vi "Read_Current_values_with_slots_select.vi"(6 "error in":errorcluster, 7 "Board_index":i32[](array[numeric])=[0, 1, 2, 3], 8 "handle":i32) -> (0 "error out":errorcluster, 1 "V0Set--I0Set":T1=[[0.0, 1.0, 0.0, 1.0, 0.0, 1.0, 0.0, 1.0], [0.0, 1.0, 0.0, 1.0, 0.0, 1.0, 0.0, 1.0], [0.0, 1.0, 0.0, 1.0, 0.0, 1.0, 0.0, 1.0], [0.0, 1.0, 0.0, 1.0, 0.0, 1.0, 0.0, 1.0], [0.0, 1.0, 0.0, 1.0, 0.0, 1.0, 0.0, 1.0], [0.0, 1.0, 0.0, 1.0, 0.0, 1.0, 0.0, 1.0], [0.0, 1.0, 0.0, 1.0, 0.0, 1.0, 0.0, 1.0], [0.0, 1.0, 0.0, 1.0, 0.0, 1.0, 0.0, 1.0], [0.0, 1.0, 0.0, 1.0, 0.0, 1.0, 0.0, 1.0], [0.0, 1.0, 0.0, 1.0, 0.0, 1.0, 0.0, 1.0], [0.0, 1.0, 0.0, 1.0, 0.0, 1.0, 0.0, 1.0], [0.0, 1.0, 0.0, 1.0, 0.0, 1.0, 0.0, 1.0]], 2 "RUp--RDWn--SVMax--Trip":T1, 3 "Status":bool[][](array[boolean]), 4 "IMon--VMon":T1, 5 "Pw":bool[][](array[boolean]))   [LabVIEW 2018]
uses:
  <vilib>/Analysis/Matrix/Datatypes/RealMatrix.ctl
  <instrlib>/CAENHVWrapper/CAENHVWrapper.lvlib
  <vilib>/Analysis/Matrix/NI_Matrix.lvlib
panel:
  # "Slot 0"
  # "Slot 1"
  # "Slot 2"
  # "Slot 3"
  # "Slot 0"
  # "Slot 1"
  # "Slot 2"
  # "Slot 3"
  # "IMon"
  # "VMon"
  # "IMon"
  # "VMon"
  # "IMon"
  # "VMon"
  # "IMon"
  # "VMon"
  # "V0Set"
  # "I0Set"
  # "V0Set"
  # "I0Set"
  # "V0Set"
  # "I0Set"
  # "V0Set"
  # "I0Set"
  # "Ch 0"
  # "Slot 0"
  # "Slot 1"
  # "Slot 2"
  # "Slot 3"
  # "Slot 0"
  # "Slot 1"
  # "Slot 2"
  # "Slot 3"
  # "Ch 0"
  # "Ch 0"
  # "Ch 1"
  # "Ch 1"
  # "Ch 1"
  # "Ch 2"
  # "Ch 2"
  # "Ch 2"
  # "Ch 3"
  # "Ch 3"
  # "Ch 3"
  # "Ch 4"
  # "Ch 4"
  # "Ch 4"
  # "Ch 5"
  # "Ch 5"
  # "Ch 5"
  # "Ch 6"
  # "Ch 6"
  # "Ch 6"
  # "Ch 7"
  # "Ch 7"
  # "Ch 7"
  # "Ch 8"
  # "Ch 8"
  # "Ch 8"
  # "Ch 9"
  # "Ch 9"
  # "Ch 9"
  # "Ch 10"
  # "Ch 10"
  # "Ch 10"
  # "Ch 11"
  # "Ch 11"
  # "Ch 11"
  # "Slot 0"
  # "Slot 1"
  # "Slot 2"
  # "Slot 3"
  # "RUp"
  # "RDWn"
  # "SVMax"
  # "Trip"
  # "RUp"
  # "RDWn"
  # "SVMax"
  # "Trip"
  # "RUp"
  # "RDWn"
  # "SVMax"
  # "Trip"
  # "RUp"
  # "RDWn"
  # "SVMax"
  # "Trip"
  # "Ch 0"
  # "Ch 1"
  # "Ch 2"
  # "Ch 3"
  # "Ch 4"
  # "Ch 5"
  # "Ch 6"
  # "Ch 7"
  # "Ch 8"
  # "Ch 9"
  # "Ch 10"
  # "Ch 11"
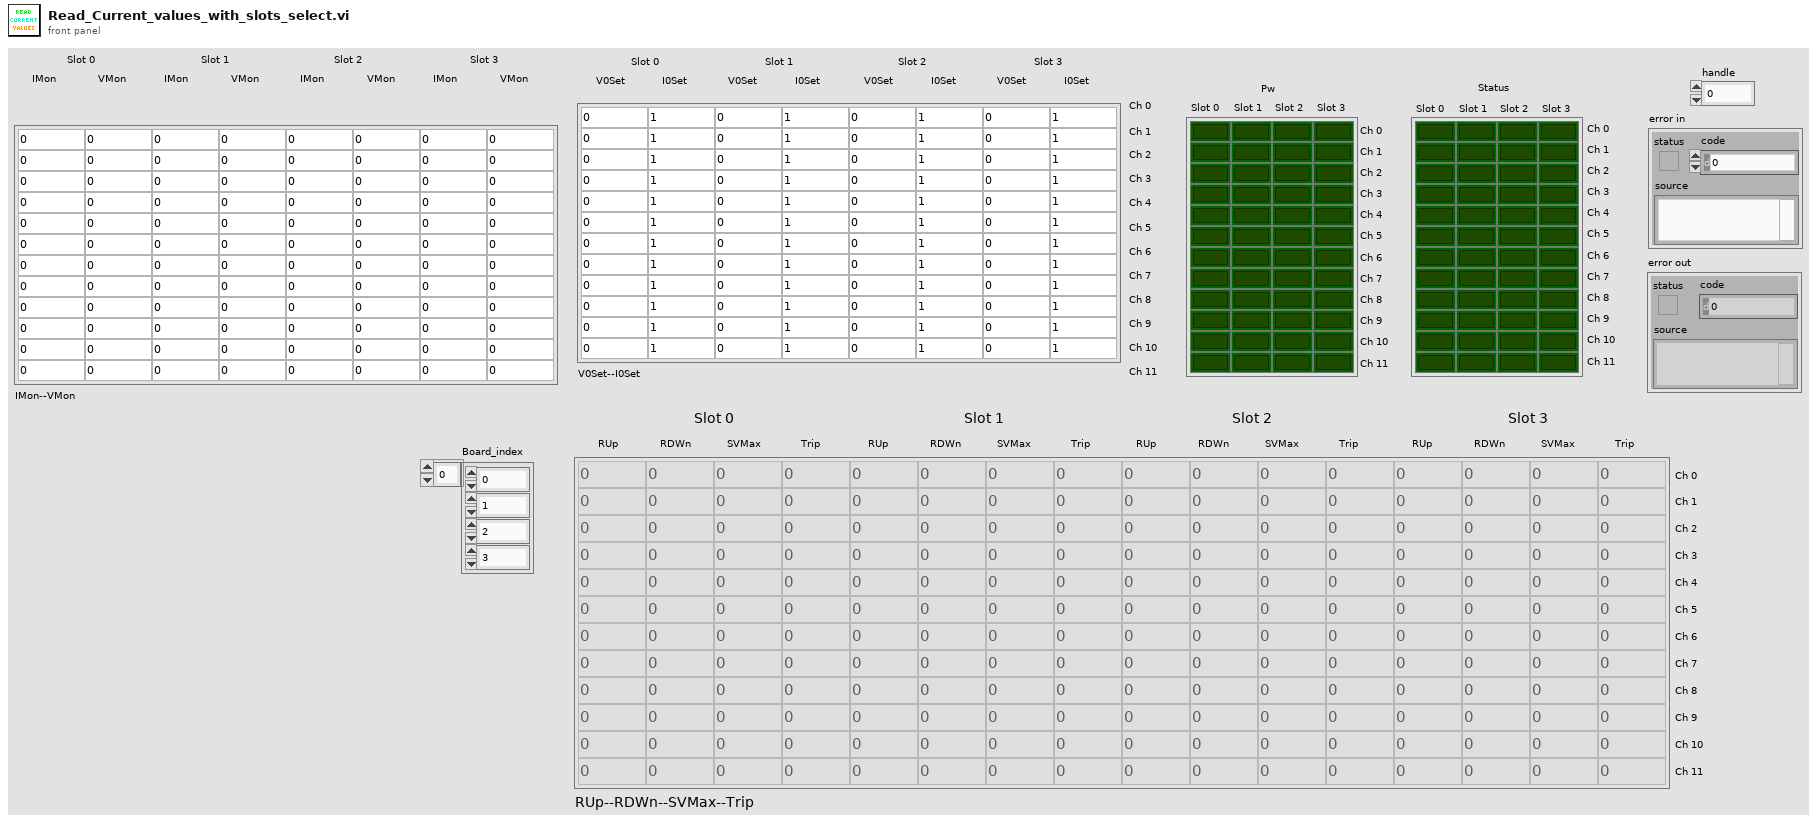
[diagram p1: front panel]
types:
  T1 = typedef "NI_Matrix.lvlib/RealMatrix.ctl" = dbl[][]
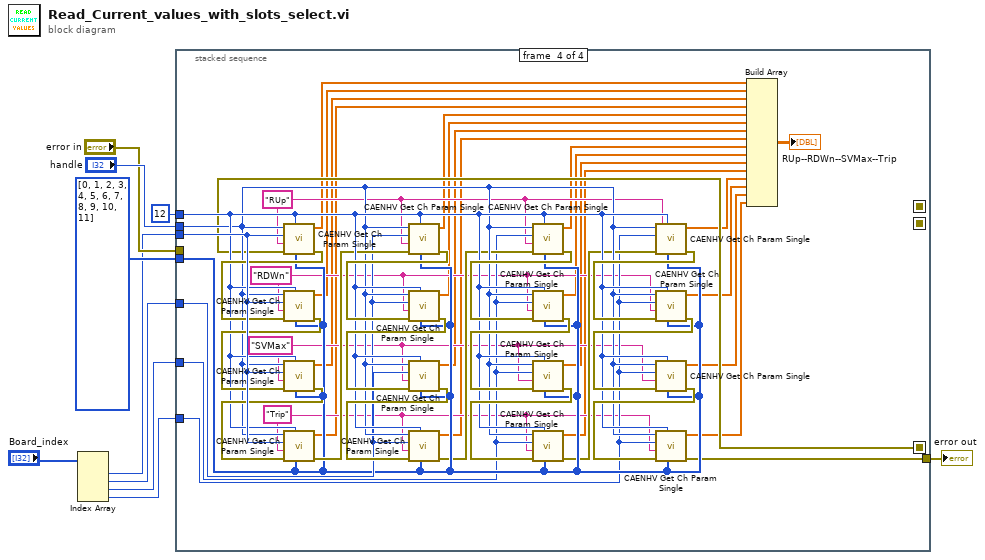
[diagram p0: block diagram]
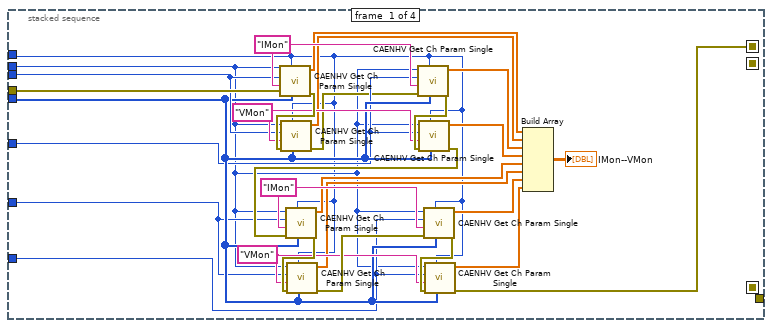
[diagram p2: hidden frame]
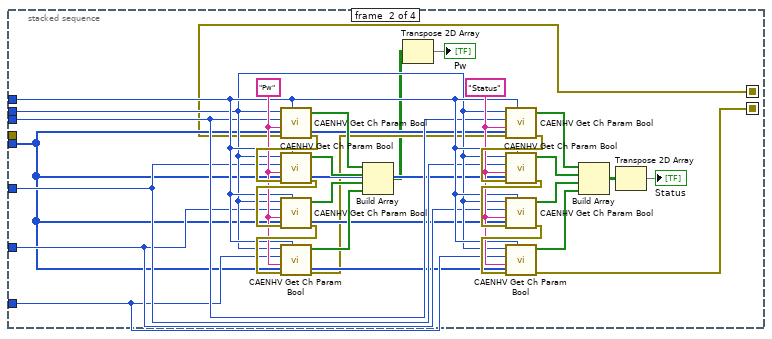
[diagram p3: hidden frame]
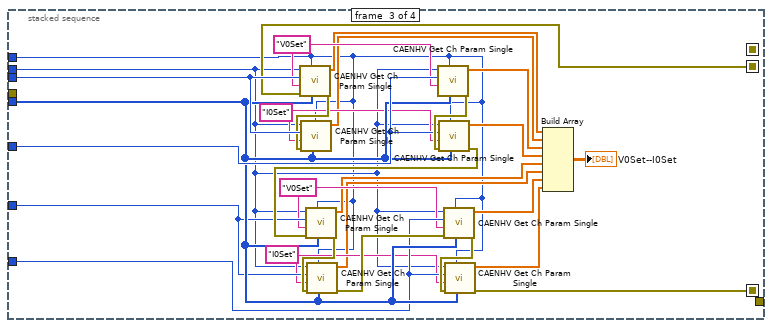
[diagram p4: hidden frame]
diagram:
  n1 = Index Array(array="Board_index") -> (element #1=w4:i32, element #2=w3:i32, element #3=w2:i32, element #4=w1:i32)  [unwired: 4 in]
  n2 = stacked-sequence {
    seq-local: [_ w45 _ _] -> [_ _ w95 _]
    seq-local: [_ _ w87 _] -> [_ _ _ w120]
    seq-local: [w14 _ _ _] -> [_ w40 _ _]
    tunnel: u16[] [0, 1, 2, 3, 4, 5, 6, 7, 8, 9, 10, 11] ("ChList") -> [w18 w47 w89 w125]
    tunnel: u16 12 ("ChNum (1)") -> [w11 w53 w70 w129]
    tunnel: "handle" -> [w12 w52 w71 w127]
    tunnel: w4 -> [w19 w51 w97 w142]
    tunnel: w3 -> [w17 w50 w93 w126]
    tunnel: w2 -> [w16 w49 w86 w123]
    tunnel: w1 -> [w15 w48 w85 w121]
    tunnel: "error in" -> [w20 _ _ _]
    tunnel: [_ _ _ w119] -> w6
    frame #0 {
      w30 = "VMon" ("y")
      w31 = "IMon" ("y")
      w32 = "VMon" ("y")
      w33 = "IMon" ("y")
      n3 = call <instrlib>:"CAENHV Get Ch Param Single.vi"("ChList"=w18, "ChNum (1)"=w11, "error in (no error)"=w20, "ParName"=w33, "slot"=w19, "handle"=w12) -> ("error out"=w39:errorcluster, "ParValList"=w28:sgl[])  [unwired: 4 in]
      n4 = call <instrlib>:"CAENHV Get Ch Param Single.vi"("ChList"=w18, "ChNum (1)"=w11, "error in (no error)"=w39, "ParName"=w32, "slot"=w19, "handle"=w12) -> ("error out"=w13:errorcluster, "ParValList"=w27:sgl[])  [unwired: 4 in]
      n5 = call <instrlib>:"CAENHV Get Ch Param Single.vi"("ChList"=w18, "ChNum (1)"=w11, "error in (no error)"=w13, "ParName"=w33, "slot"=w17, "handle"=w12) -> ("error out"=w38:errorcluster, "ParValList"=w26:sgl[])  [unwired: 4 in]
      n6 = call <instrlib>:"CAENHV Get Ch Param Single.vi"("ChList"=w18, "ChNum (1)"=w11, "error in (no error)"=w38, "ParName"=w32, "slot"=w17, "handle"=w12) -> ("error out"=w35:errorcluster, "ParValList"=w25:sgl[])  [unwired: 4 in]
      n7 = call <instrlib>:"CAENHV Get Ch Param Single.vi"("ChList"=w18, "ChNum (1)"=w11, "error in (no error)"=w35, "ParName"=w31, "slot"=w16, "handle"=w12) -> ("error out"=w36:errorcluster, "ParValList"=w24:sgl[])  [unwired: 4 in]
      n8 = call <instrlib>:"CAENHV Get Ch Param Single.vi"("ChList"=w18, "ChNum (1)"=w11, "error in (no error)"=w36, "ParName"=w30, "slot"=w16, "handle"=w12) -> ("error out"=w34:errorcluster, "ParValList"=w23:sgl[])  [unwired: 4 in]
      n9 = call <instrlib>:"CAENHV Get Ch Param Single.vi"("ChList"=w18, "ChNum (1)"=w11, "error in (no error)"=w34, "ParName"=w31, "slot"=w15, "handle"=w12) -> ("error out"=w37:errorcluster, "ParValList"=w22:sgl[])  [unwired: 4 in]
      n10 = call <instrlib>:"CAENHV Get Ch Param Single.vi"("ChList"=w18, "ChNum (1)"=w11, "error in (no error)"=w37, "ParName"=w30, "slot"=w15, "handle"=w12) -> ("error out"=w14:errorcluster, "ParValList"=w21:sgl[])  [unwired: 4 in]
      n11 = Build Array(w28, w27, w26, w25, w24, w23, w22, w21) -> (→"IMon--VMon":T1)
    }
    frame #1 {
      w58 = "Status" ("y")
      w66 = "Pw" ("y")
      n12 = call <instrlib>:"CAENHV Get Ch Param Bool.vi"("ChList"=w47, "ChNum (1)"=w53, "error in (no error)"=w40, "ParName"=w66, "slot"=w51, "handle"=w52) -> ("error out"=w69:errorcluster, "ParValList"=w65:bool[])  [unwired: 4 in]
      n13 = call <instrlib>:"CAENHV Get Ch Param Bool.vi"("ChList"=w47, "ChNum (1)"=w53, "error in (no error)"=w69, "ParName"=w66, "slot"=w50, "handle"=w52) -> ("error out"=w68:errorcluster, "ParValList"=w64:bool[])  [unwired: 4 in]
      n14 = call <instrlib>:"CAENHV Get Ch Param Bool.vi"("ChList"=w47, "ChNum (1)"=w53, "error in (no error)"=w68, "ParName"=w66, "slot"=w49, "handle"=w52) -> ("error out"=w67:errorcluster, "ParValList"=w63:bool[])  [unwired: 4 in]
      n15 = call <instrlib>:"CAENHV Get Ch Param Bool.vi"("ChList"=w47, "ChNum (1)"=w53, "error in (no error)"=w67, "ParName"=w66, "slot"=w48, "handle"=w52) -> ("error out"=w46:errorcluster, "ParValList"=w62:bool[])  [unwired: 4 in]
      n16 = Build Array(w65, w64, w63, w62) -> (w44:bool[][])
      n17 = Transpose 2D Array(2D array=w44) -> (transposed array=→"Pw":bool[][])
      n18 = call <instrlib>:"CAENHV Get Ch Param Bool.vi"("ChList"=w47, "ChNum (1)"=w53, "error in (no error)"=w46, "ParName"=w58, "slot"=w51, "handle"=w52) -> ("error out"=w61:errorcluster, "ParValList"=w57:bool[])  [unwired: 4 in]
      n19 = call <instrlib>:"CAENHV Get Ch Param Bool.vi"("ChList"=w47, "ChNum (1)"=w53, "error in (no error)"=w61, "ParName"=w58, "slot"=w50, "handle"=w52) -> ("error out"=w60:errorcluster, "ParValList"=w56:bool[])  [unwired: 4 in]
      n20 = call <instrlib>:"CAENHV Get Ch Param Bool.vi"("ChList"=w47, "ChNum (1)"=w53, "error in (no error)"=w60, "ParName"=w58, "slot"=w49, "handle"=w52) -> ("error out"=w59:errorcluster, "ParValList"=w55:bool[])  [unwired: 4 in]
      n21 = call <instrlib>:"CAENHV Get Ch Param Bool.vi"("ChList"=w47, "ChNum (1)"=w53, "error in (no error)"=w59, "ParName"=w58, "slot"=w48, "handle"=w52) -> ("error out"=w45:errorcluster, "ParValList"=w54:bool[])  [unwired: 4 in]
      n22 = Build Array(w57, w56, w55, w54) -> (w42:bool[][])
      n23 = Transpose 2D Array(2D array=w42) -> (transposed array=→"Status":bool[][])
    }
    frame #2 {
      w81 = "I0Set" ("y")
      w82 = "V0Set" ("y")
      w83 = "I0Set" ("y")
      w84 = "V0Set" ("y")
      n24 = call <instrlib>:"CAENHV Get Ch Param Single.vi"("ChList"=w89, "ChNum (1)"=w70, "error in (no error)"=w95, "ParName"=w84, "slot"=w97, "handle"=w71) -> ("error out"=w96:errorcluster, "ParValList"=w79:sgl[])  [unwired: 4 in]
      n25 = call <instrlib>:"CAENHV Get Ch Param Single.vi"("ChList"=w89, "ChNum (1)"=w70, "error in (no error)"=w96, "ParName"=w83, "slot"=w97, "handle"=w71) -> ("ParValList"=w78:sgl[])  [unwired: 4 in, 1 out]
      n26 = call <instrlib>:"CAENHV Get Ch Param Single.vi"("ChList"=w89, "ChNum (1)"=w70, "ParName"=w84, "slot"=w93, "handle"=w71) -> ("error out"=w94:errorcluster, "ParValList"=w77:sgl[])  [unwired: 5 in]
      n27 = call <instrlib>:"CAENHV Get Ch Param Single.vi"("ChList"=w89, "ChNum (1)"=w70, "error in (no error)"=w94, "ParName"=w83, "slot"=w93, "handle"=w71) -> ("error out"=w90:errorcluster, "ParValList"=w76:sgl[])  [unwired: 4 in]
      n28 = call <instrlib>:"CAENHV Get Ch Param Single.vi"("ChList"=w89, "ChNum (1)"=w70, "error in (no error)"=w90, "ParName"=w82, "slot"=w86, "handle"=w71) -> ("error out"=w91:errorcluster, "ParValList"=w75:sgl[])  [unwired: 4 in]
      n29 = call <instrlib>:"CAENHV Get Ch Param Single.vi"("ChList"=w89, "ChNum (1)"=w70, "error in (no error)"=w91, "ParName"=w81, "slot"=w86, "handle"=w71) -> ("error out"=w88:errorcluster, "ParValList"=w74:sgl[])  [unwired: 4 in]
      n30 = call <instrlib>:"CAENHV Get Ch Param Single.vi"("ChList"=w89, "ChNum (1)"=w70, "error in (no error)"=w88, "ParName"=w82, "slot"=w85, "handle"=w71) -> ("error out"=w92:errorcluster, "ParValList"=w73:sgl[])  [unwired: 4 in]
      n31 = call <instrlib>:"CAENHV Get Ch Param Single.vi"("ChList"=w89, "ChNum (1)"=w70, "error in (no error)"=w92, "ParName"=w81, "slot"=w85, "handle"=w71) -> ("error out"=w87:errorcluster, "ParValList"=w72:sgl[])  [unwired: 4 in]
      n32 = Build Array(w79, w78, w77, w76, w75, w74, w73, w72) -> (→"V0Set--I0Set":T1)
    }
    frame #3 {
      w115 = "Trip" ("y")
      w116 = "SVMax" ("y")
      w118 = "RDWn" ("y")
      w117 = "RUp" ("y")
      n33 = call <instrlib>:"CAENHV Get Ch Param Single.vi"("ChList"=w125, "ChNum (1)"=w129, "error in (no error)"=w120, "ParName"=w117, "slot"=w142, "handle"=w127) -> ("error out"=w141:errorcluster, "ParValList"=w113:sgl[])  [unwired: 4 in]
      n34 = call <instrlib>:"CAENHV Get Ch Param Single.vi"("ChList"=w125, "ChNum (1)"=w129, "error in (no error)"=w141, "ParName"=w118, "slot"=w142, "handle"=w127) -> ("error out"=w140:errorcluster, "ParValList"=w112:sgl[])  [unwired: 4 in]
      n35 = call <instrlib>:"CAENHV Get Ch Param Single.vi"("ChList"=w125, "ChNum (1)"=w129, "error in (no error)"=w140, "ParName"=w116, "slot"=w142, "handle"=w127) -> ("error out"=w139:errorcluster, "ParValList"=w111:sgl[])  [unwired: 4 in]
      n36 = call <instrlib>:"CAENHV Get Ch Param Single.vi"("ChList"=w125, "ChNum (1)"=w129, "error in (no error)"=w139, "ParName"=w115, "slot"=w142, "handle"=w127) -> ("error out"=w128:errorcluster, "ParValList"=w110:sgl[])  [unwired: 4 in]
      n37 = call <instrlib>:"CAENHV Get Ch Param Single.vi"("ChList"=w125, "ChNum (1)"=w129, "error in (no error)"=w128, "ParName"=w117, "slot"=w126, "handle"=w127) -> ("error out"=w136:errorcluster, "ParValList"=w109:sgl[])  [unwired: 4 in]
      n38 = call <instrlib>:"CAENHV Get Ch Param Single.vi"("ChList"=w125, "ChNum (1)"=w129, "error in (no error)"=w136, "ParName"=w118, "slot"=w126, "handle"=w127) -> ("error out"=w137:errorcluster, "ParValList"=w108:sgl[])  [unwired: 4 in]
      n39 = call <instrlib>:"CAENHV Get Ch Param Single.vi"("ChList"=w125, "ChNum (1)"=w129, "error in (no error)"=w137, "ParName"=w116, "slot"=w126, "handle"=w127) -> ("error out"=w138:errorcluster, "ParValList"=w107:sgl[])  [unwired: 4 in]
      n40 = call <instrlib>:"CAENHV Get Ch Param Single.vi"("ChList"=w125, "ChNum (1)"=w129, "error in (no error)"=w138, "ParName"=w115, "slot"=w126, "handle"=w127) -> ("error out"=w124:errorcluster, "ParValList"=w106:sgl[])  [unwired: 4 in]
      n41 = call <instrlib>:"CAENHV Get Ch Param Single.vi"("ChList"=w125, "ChNum (1)"=w129, "error in (no error)"=w124, "ParName"=w117, "slot"=w123, "handle"=w127) -> ("error out"=w135:errorcluster, "ParValList"=w105:sgl[])  [unwired: 4 in]
      n42 = call <instrlib>:"CAENHV Get Ch Param Single.vi"("ChList"=w125, "ChNum (1)"=w129, "error in (no error)"=w135, "ParName"=w118, "slot"=w123, "handle"=w127) -> ("error out"=w134:errorcluster, "ParValList"=w104:sgl[])  [unwired: 4 in]
      n43 = call <instrlib>:"CAENHV Get Ch Param Single.vi"("ChList"=w125, "ChNum (1)"=w129, "error in (no error)"=w134, "ParName"=w116, "slot"=w123, "handle"=w127) -> ("error out"=w133:errorcluster, "ParValList"=w103:sgl[])  [unwired: 4 in]
      n44 = call <instrlib>:"CAENHV Get Ch Param Single.vi"("ChList"=w125, "ChNum (1)"=w129, "error in (no error)"=w133, "ParName"=w115, "slot"=w123, "handle"=w127) -> ("error out"=w122:errorcluster, "ParValList"=w102:sgl[])  [unwired: 4 in]
      n45 = call <instrlib>:"CAENHV Get Ch Param Single.vi"("ChList"=w125, "ChNum (1)"=w129, "error in (no error)"=w122, "ParName"=w117, "slot"=w121, "handle"=w127) -> ("error out"=w130:errorcluster, "ParValList"=w101:sgl[])  [unwired: 4 in]
      n46 = call <instrlib>:"CAENHV Get Ch Param Single.vi"("ChList"=w125, "ChNum (1)"=w129, "error in (no error)"=w130, "ParName"=w118, "slot"=w121, "handle"=w127) -> ("error out"=w131:errorcluster, "ParValList"=w100:sgl[])  [unwired: 4 in]
      n47 = call <instrlib>:"CAENHV Get Ch Param Single.vi"("ChList"=w125, "ChNum (1)"=w129, "error in (no error)"=w131, "ParName"=w116, "slot"=w121, "handle"=w127) -> ("error out"=w132:errorcluster, "ParValList"=w99:sgl[])  [unwired: 4 in]
      n48 = call <instrlib>:"CAENHV Get Ch Param Single.vi"("ChList"=w125, "ChNum (1)"=w129, "error in (no error)"=w132, "ParName"=w115, "slot"=w121, "handle"=w127) -> ("error out"=w119:errorcluster, "ParValList"=w98:sgl[])  [unwired: 4 in]
      n49 = Build Array(w113, w112, w111, w110, w109, w108, w107, w106, w105, w104, w103, w102, w101, w100, w99, w98) -> (→"RUp--RDWn--SVMax--Trip":T1)
    }
  }
  "error out" <- w6
